vi "Joystick 2 ClimbSystem.vi"(9 "Range of motion":dbl=90.0 format="%#_13g", 10 "Secondary Joystick Buttons":bool[](array[boolean]), 11 "Secondary Joystick Values":dbl[](array[numeric])) -> (2 "Reset Climber Encoder":bool, 3 "Desired Climber Angle":dbl)   [LabVIEW 2018]
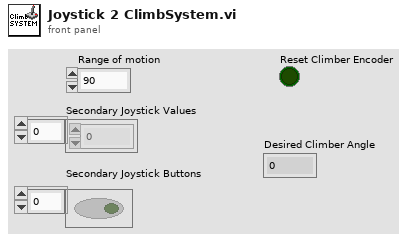
[diagram p1: front panel]
types:
  T1 = typedef "SecondaryJoystickButtons.ctl" = cluster{"Intake":bool, "Outtake":bool, "Arm Up":bool, "Arm Down":bool, "Open Grip":bool, "Close Grip":bool, "Climber Up":bool, "Climber Down":bool, "Reset Climber Encoder":bool}
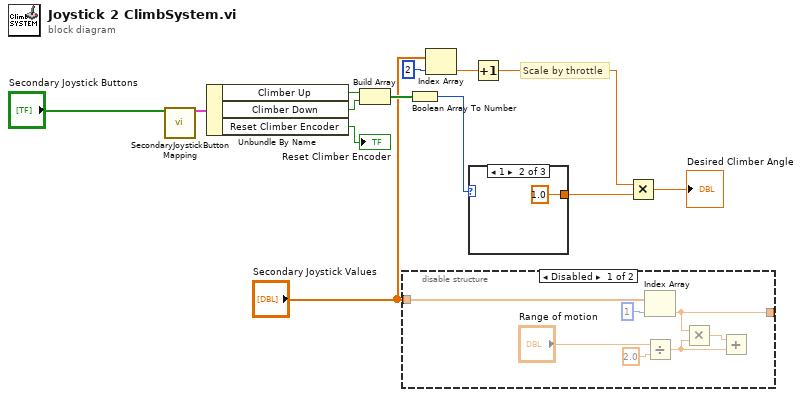
[diagram p0: block diagram]
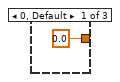
[diagram p2: hidden frame]
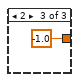
[diagram p3: hidden frame]
diagram:
  # "Scale by throttle"
  n1 = call "SecondaryJoystickButtonMapping.vi"("Secondary joystick buttons"="Secondary Joystick Buttons") -> ("SecondaryJoystickButtons"=w12:T1)  [unwired: 13 in, 1 out]
  n2 = Unbundle By Name(w12) -> ("Climber Up"=w10:bool, "Climber Down"=w9:bool, "Reset Climber Encoder"=→"Reset Climber Encoder":bool)
  n3 = Build Array(w10, w9) -> (w8:bool[])
  n4 = disable-structure shown="Disabled" {
    disable-tunnel: [w15 _] -> _
    disable-tunnel: "Secondary Joystick Values" -> [w14 _]
    frame Disabled {
      n5 = Index Array(array=w14, index=1) -> (element=w15:dbl)
      n6 = Divide(x="Range of motion", y=2.0) -> (x/y=w17:dbl)
      n7 = Multiply(x=w15, y=w17) -> (x*y=w19:dbl)
      n8 = Add(x=w19, y=w17) -> ()  [unwired: 1 out]
    }
    frame Enabled {
    }
  }
  n9 = Boolean Array To Number(Boolean array=w8) -> (number=w7:u32)
  n10 = Index Array(array="Secondary Joystick Values", index=2) -> (element=w2:dbl)
  n11 = case shown="1" w7 {
    tunnel: [0.0 1.0 -1.0] -> w6
    frame 0, Default {
    }
    frame 1 {
    }
    frame 2 {
    }
  }
  n12 = Increment(x=w2) -> (x+1=w1:dbl)
  n13 = Multiply(x=w1, y=w6) -> (x*y=→"Desired Climber Angle":dbl)
